vi "Keithley 2450 Sweep and Acquire Measurements.vi"() -> ()   [LabVIEW 2021]
doc: "Configures a sweep and takes voltage and current readings at each point."
uses:
  <instrlib>/Keithley 2450/Public/Data/Read (Multiple Points).vi
  <instrlib>/Keithley 2450/Keithley 2450.lvlib
panel:
  in  "Limit Level (0.1)":dbl=0.1
  in  "Delay (0) in Sec":dbl
  in  "Measurement Speed (1 PLC)":dbl=1.0 format="%.2g"
  in  "Sweep Points":T1={"Start "=1.0, "Stop "=0.0, "Number of Points (5)"=5}
  in  "Source Mode  (0: Voltage)":u16(ring) items=["Voltage", "Current"]
  in  "VISA resource name":refnum<visa-resource-name>
  out "Waveform Graph":dbl[][](graph)
  # "(c) 2021 National Instruments.  ALL RIGHTS RESERVED."
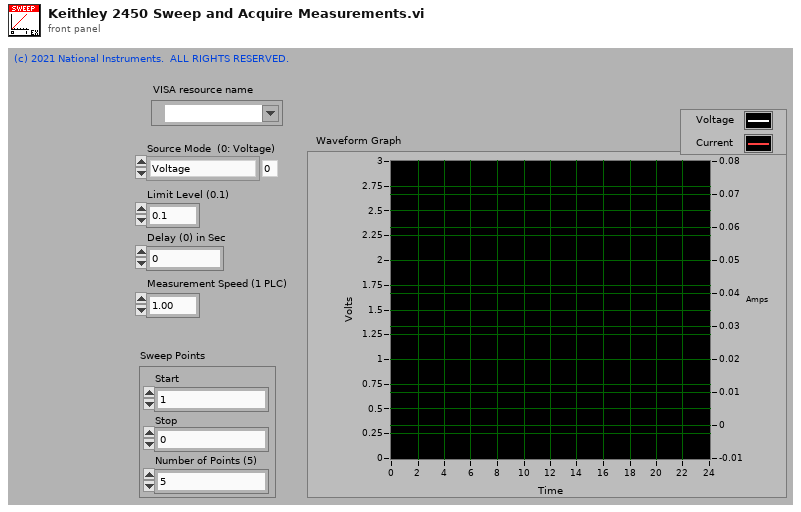
[diagram p1: front panel]
types:
  T1 = cluster{"Start ":dbl, "Stop ":dbl, "Number of Points (5)":u32}
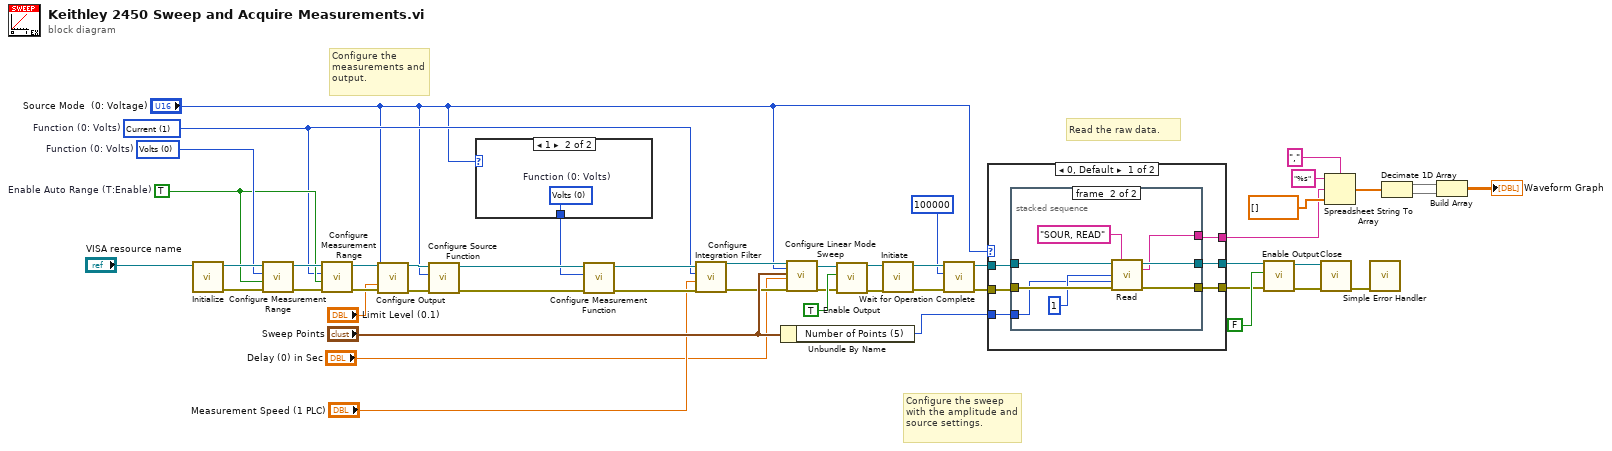
[diagram p0: block diagram]
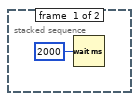
[diagram p2: hidden frame]
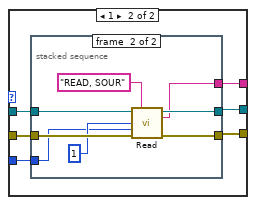
[diagram p3: hidden frame]
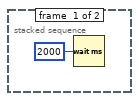
[diagram p4: hidden frame]
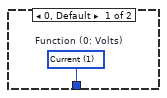
[diagram p5: hidden frame]
diagram:
  w39 = TRUE  # Enable Auto Range (T:Enable)
  w12 = u16 1 items=["Volts", "Current", "Resistance"]  # Function (0: Volts)
  w40 = u16 0 items=["Volts", "Current", "Resistance"]  # Function (0: Volts)
  # "Read the raw data."
  # "Configure the sweep with the amplitude and source settings."
  # "Configure the measurements and output."
  n1 = call <instrlib>:"Initialize.vi"("VISA resource name"="VISA resource name") -> ("error out"=w48:errorcluster, "VISA resource name out"=w49:refnum<visa-resource-name>)  [unwired: 9 in]
  n2 = call <instrlib>:"Configure Measurement Range.vi"("error in (no error)"=w48, "Enable Auto Range (T:Enable)"=w39, "Function (0: Volts)"=w40, "VISA resource name"=w49) -> ("error out"=w47:errorcluster, "VISA resource name out"=w46:refnum<visa-resource-name>)  [unwired: 6 in]
  n3 = call <instrlib>:"Configure Measurement Range.vi"("error in (no error)"=w47, "Enable Auto Range (T:Enable)"=w39, "Function (0: Volts)"=w12, "VISA resource name"=w46) -> ("error out"=w36:errorcluster, "VISA resource name out"=w37:refnum<visa-resource-name>)  [unwired: 6 in]
  n4 = call <instrlib>:"Configure Output.vi"("VISA resource name"=w37, "Source Mode  (0: Voltage)"="Source Mode  (0: Voltage)", "Source Limit Level (0.1)"="Limit Level (0.1)", "error in (no error)"=w36) -> ("VISA resource name out"=w34:refnum<visa-resource-name>, "error out"=w35:errorcluster)  [unwired: 10 in]
  n5 = call <instrlib>:"Configure Source Function.vi"("error in (no error)"=w35, "Function (0: Volts)"="Source Mode  (0: Voltage)", "VISA resource name"=w34) -> ("error out"=w15:errorcluster, "VISA resource name out"=w16:refnum<visa-resource-name>)  [unwired: 7 in]
  n6 = case shown="1" "Source Mode  (0: Voltage)" {
    tunnel: [w50 w51] -> w11
    frame 0, Default {
      w50 = u16 1 items=["Volts", "Current", "Resistance"]  # Function (0: Volts)
    }
    frame 1 {
      w51 = u16 0 items=["Volts", "Current", "Resistance"]  # Function (0: Volts)
    }
  }
  n7 = call <instrlib>:"Configure Measurement Function.vi"("error in (no error)"=w15, "Function (0: Volts)"=w11, "VISA resource name"=w16) -> ("error out"=w14:errorcluster, "VISA resource name out"=w13:refnum<visa-resource-name>)  [unwired: 7 in]
  n8 = call <instrlib>:"Configure Integration Filter.vi"("error in (no error)"=w14, "Measurement Speed (1 PLC)"="Measurement Speed (1 PLC)", "Function (0: Volts)"=w12, "VISA resource name"=w13) -> ("error out"=w19:errorcluster, "VISA resource name out"=w18:refnum<visa-resource-name>)  [unwired: 6 in]
  n9 = Unbundle By Name("Sweep Points") -> ("Number of Points (5)"=w5:u32)
  n10 = call <instrlib>:"Configure Linear Mode Sweep.vi"("VISA resource name"=w18, "Source Mode  (0: Voltage)"="Source Mode  (0: Voltage)", "Sweep Points"="Sweep Points", "Delay (0)"="Delay (0) in Sec", "error in (no error)"=w19) -> ("VISA resource name out"=w33:refnum<visa-resource-name>, "error out"=w32:errorcluster)  [unwired: 13 in]
  n11 = call <instrlib>:"Enable Output.vi"("error in (no error)"=w32, "Enable Output (T: Enable)"=TRUE, "VISA resource name"=w33) -> ("error out"=w30:errorcluster, "VISA resource name out"=w31:refnum<visa-resource-name>)  [unwired: 7 in]
  n12 = call <instrlib>:"Initiate.vi"("error in (no error)"=w30, "VISA resource name"=w31) -> ("error out"=w20:errorcluster, "VISA resource name out"=w21:refnum<visa-resource-name>)  [unwired: 8 in]
  n13 = call <instrlib>:"Wait for Operation Complete.vi"("error in (no error)"=w20, "Timeout (10000 ms)"=100000, "VISA resource name"=w21) -> ("error out"=w8:errorcluster, "VISA resource name out"=w9:refnum<visa-resource-name>)  [unwired: 7 in]
  n14 = case shown="0, Default" "Source Mode  (0: Voltage)" {
    tunnel: w9 -> [w57 w72]
    tunnel: w8 -> [w56 w71]
    tunnel: [w55 w69] -> w7
    tunnel: [w54 w68] -> w6
    tunnel: w5 -> [w53 w70]
    tunnel: [w52 w67] -> w4
    frame 0, Default {
      n15 = stacked-sequence {
        tunnel: [_ w66] -> w55
        tunnel: [_ w65] -> w54
        tunnel: w57 -> [_ w63]
        tunnel: w56 -> [_ w62]
        tunnel: [_ w61] -> w52
        tunnel: w53 -> [_ w59]
        frame #0 {
          n16 = Wait (ms)(milliseconds to wait=u32 2000) -> ()  [unwired: 1 out]
        }
        frame #1 {
          n17 = call-poly <instrlib>:"Read.vi"("VISA resource name"=w63, "Buffer Elements"="SOUR, READ", "Start Index (1)"=1, "End Index (1)"=w59, "error in (no error)"=w62) -> ("VISA resource name out"=w66:refnum<visa-resource-name>, "Data out"=w61:string, "error out"=w65:errorcluster)  [unwired: 8 in]
        }
      }
    }
    frame 1 {
      n18 = stacked-sequence {
        tunnel: [_ w81] -> w69
        tunnel: [_ w80] -> w68
        tunnel: w72 -> [_ w78]
        tunnel: w71 -> [_ w77]
        tunnel: [_ w76] -> w67
        tunnel: w70 -> [_ w74]
        frame #0 {
          n19 = Wait (ms)(milliseconds to wait=u32 2000) -> ()  [unwired: 1 out]
        }
        frame #1 {
          n20 = call-poly <instrlib>:"Read.vi"("VISA resource name"=w78, "Buffer Elements"="READ, SOUR", "Start Index (1)"=1, "End Index (1)"=w74, "error in (no error)"=w77) -> ("VISA resource name out"=w81:refnum<visa-resource-name>, "Data out"=w76:string, "error out"=w80:errorcluster)  [unwired: 8 in]
        }
      }
    }
  }
  n21 = call <instrlib>:"Enable Output.vi"("error in (no error)"=w6, "Enable Output (T: Enable)"=FALSE, "VISA resource name"=w7) -> ("error out"=w42:errorcluster, "VISA resource name out"=w43:refnum<visa-resource-name>)  [unwired: 7 in]
  n22 = call <instrlib>:"Close.vi"("error in (no error)"=w42, "VISA resource name"=w43) -> ("error out"=w44:errorcluster)  [unwired: 9 in]
  n23 = Spreadsheet String To Array(delimiter (Tab)=",", format string="%s", spreadsheet string=w4, array type (2D Dbl)=dbl[] []) -> (array=w25:dbl[])
  n24 = call <vilib>:"Simple Error Handler.vi"("error in (no error)"=w44) -> ()  [unwired: 4 in, 5 out]
  n25 = Decimate 1D Array(w25) -> (w24:dbl[], w23:dbl[])
  n26 = Build Array(w24, w23) -> (→"Waveform Graph":dbl[][])
